vi "Set Drawing Style.vi"(5 "Face Culling Mode":T1(ring), 7 "Frontface Mode":T2(ring), 8 "error in (no error)":errorcluster, 9 "Size":dbl=-1.0, 10 "Mode":T3(ring)=enum."Polygons", 11 "Scene Object In":refnum<vi>) -> (0 "error out":errorcluster, 3 "Scene Object Out":refnum<vi>)   [LabVIEW 2020, in "NI_3D Picture Control.lvlib"]
doc: "Specifies the rendering mode for 3D objects."
uses:
  <vilib>/picture/3D Picture Control/NI_3D Picture Control.lvlib
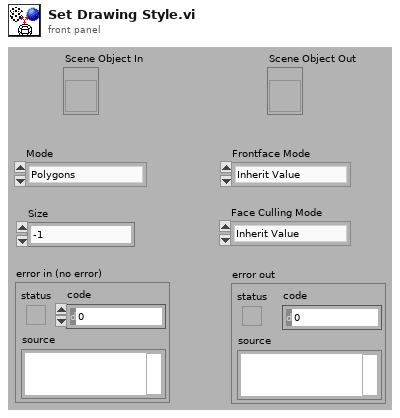
[diagram p1: front panel]
types:
  T1 = enum16{"Inherit Value", "No Culling", "Cull Back Face", "Cull Front Face", "Cull Both Faces"}
  T2 = enum16{"Inherit Value", "Counterclockwise", "Clockwise"}
  T3 = enum16{"Inherit Value", "Points", "Wireframe", "Polygons"}
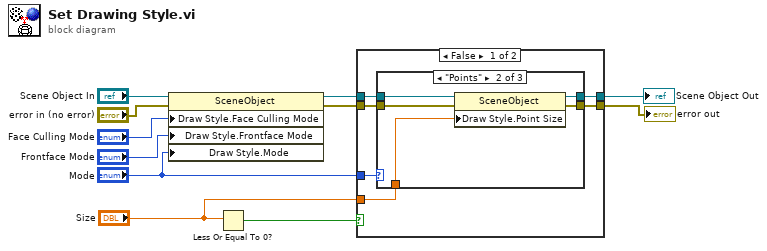
[diagram p0: block diagram]
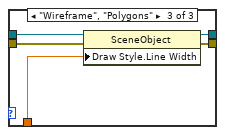
[diagram p3: hidden frame]
diagram:
  n1 = property class="SceneObject"(reference="Scene Object In", error in="error in (no error)", "Draw Style.Face Culling Mode"="Face Culling Mode", "Draw Style.Frontface Mode"="Frontface Mode", "Draw Style.Mode"="Mode") -> (reference out=w5:refnum<vi>, error out=w3:errorcluster)
  n2 = Less Or Equal To 0?(x="Size") -> (x <= 0?=w7:bool)
  n3 = case shown="False" w7 {
    tunnel: [w17 w31] -> w6
    tunnel: w5 -> [w16 w31]
    tunnel: [w12 w30] -> w4
    tunnel: w3 -> [w13 w30]
    tunnel: "Mode" -> [w15 _]
    tunnel: "Size" -> [w14 _]
    frame False {
      n4 = case shown="\"Points\"" w15 {
        tunnel: [w19 w24 w29] -> w17
        tunnel: w16 -> [w19 w23 w28]
        tunnel: w14 -> [_ w22 w27]
        tunnel: w13 -> [w18 w21 w26]
        tunnel: [w18 w20 w25] -> w12
        frame "Inherit Value" {
        }
        frame "Points" {
          n5 = property class="SceneObject"(reference=w23, error in=w21, "Draw Style.Point Size"=w22) -> (reference out=w24:refnum<vi>, error out=w20:errorcluster)
        }
        frame "Wireframe", "Polygons" {
          n6 = property class="SceneObject"(reference=w28, error in=w26, "Draw Style.Line Width"=w27) -> (reference out=w29:refnum<vi>, error out=w25:errorcluster)
        }
      }
    }
    frame True {
    }
  }
  "Scene Object Out" <- w6
  "error out" <- w4
